vi "CheckReferenceValue.vi"(10 "YCoordIn":sgl format="%#_13g", 11 "XCoordIn":sgl format="%#_13g") -> (0 "YCoordCorrect":bool, 1 "XCoordCorrect":bool, 2 "YCoordOut":sgl format="%#_13g", 3 "XCoordOut":sgl format="%#_13g")   [LabVIEW 2017]
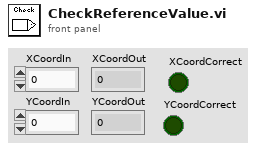
[diagram p1: front panel]
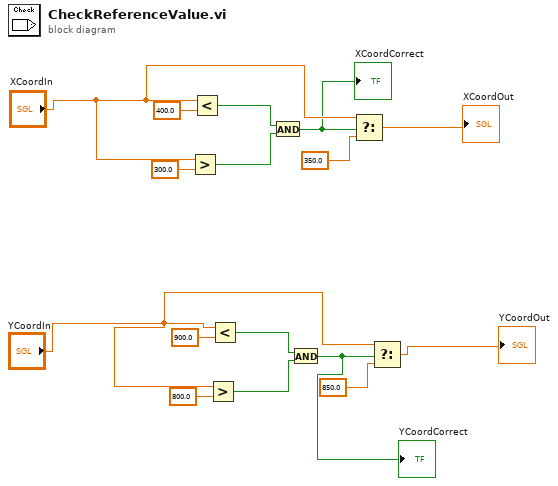
[diagram p0: block diagram]
diagram:
  n1 = Greater?(x="XCoordIn", y=sgl 300.0) -> (0:w15:bool)
  n2 = Less?(x="XCoordIn", y=sgl 400.0) -> (x < y?=w16:bool)
  n3 = Greater?(x="YCoordIn", y=sgl 800.0) -> (0:w8:bool)
  n4 = Less?(x="YCoordIn", y=sgl 900.0) -> (x < y?=w9:bool)
  n5 = And(x=w16, y=w15) -> (x .and. y?=w2:bool)
  "XCoordCorrect" <- w2
  n6 = And(x=w9, y=w8) -> (x .and. y?=w1:bool)
  "YCoordCorrect" <- w1
  n7 = Select(t="XCoordIn", s=w2, f=sgl 350.0 ("y")) -> (s? t:f=→"XCoordOut":sgl)
  n8 = Select(t="YCoordIn", s=w1, f=sgl 850.0 ("y")) -> (s? t:f=→"YCoordOut":sgl)
